vi "dvp Vi Get Color Temperature State.vi"(10 "pColorTemperatureState":i32, 11 "handle":u32) -> (2 "pColorTemperatureState out":i32, 3 "function return":u32(ring))   [LabVIEW 2018, in "LabViewDVPCamera.lvlib"]
doc: "LabviewDvp2Api dvpStatus dvpViGetColorTemperatureState(dvpHandle handle, BOOL *pColorTemperatureState);"
uses:
  LabViewDVPCamera.lvlib
  LabViewDVPCamera/LabViewDVPCamera.dll
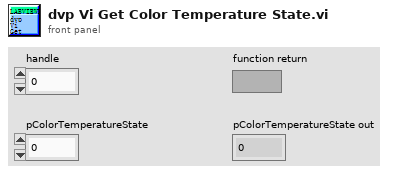
[diagram p1: front panel]
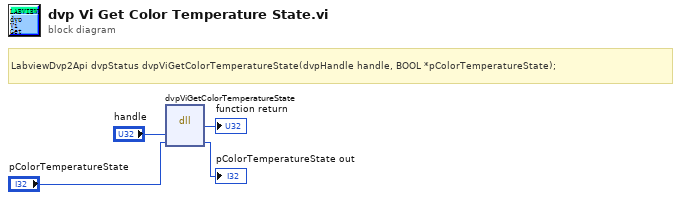
[diagram p0: block diagram]
diagram:
  # "LabviewDvp2Api dvpStatus dvpViGetColorTemperatureState(dvpHandle handle, BOOL *pColorTemperatureState);"
  n1 = dll-call lib="C:/Program Files (x86)/DVP2 Labview cn 64/Sample/LabViewDVPCamera/LabViewDVPCamera.*" fn="dvpViGetColorTemperatureState"("handle"="handle", "pColorTemperatureState"="pColorTemperatureState") -> (→"function return":u32, "pColorTemperatureState"=→"pColorTemperatureState out":i32)  [unwired: 4 in, 2 out]
